vi "OpenSubVIS.vi"(8 "error in (no error)":errorcluster caption="错误输入（无错误）", 10 "自动关闭前面板？":bool, 11 "路径或VI名称":path) -> (0 "error out":errorcluster caption="错误输出")   [LabVIEW 2018]
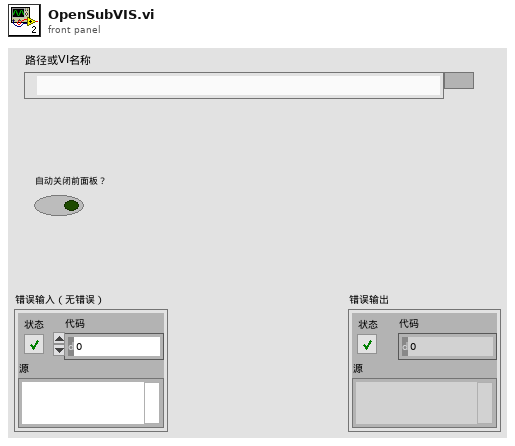
[diagram p1: front panel]
types:
  T1 = enum32{"Bad", "Idle", "Run top level", "Running"}
  T2 = enum32{"Invalid", "Standard", "Closed", "Hidden", "Minimized", "Maximized"}
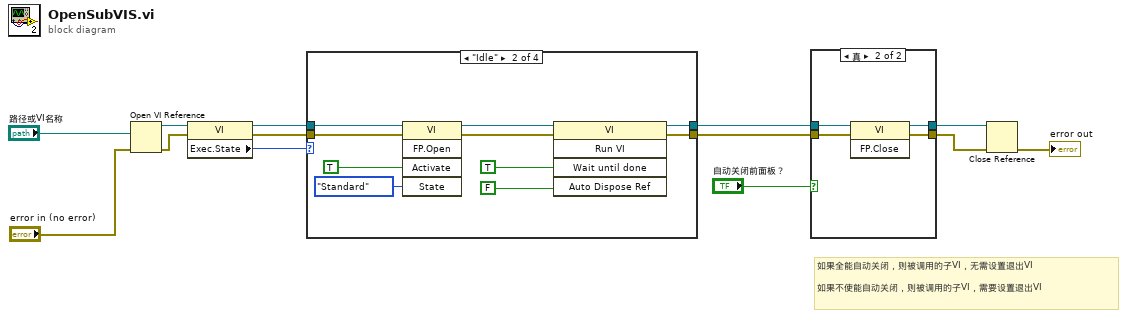
[diagram p0: block diagram]
diagram:
  # "如果全能自动关闭，则被调用的子VI，无需设置退出VI\n\n如果不使能自动关闭，则被调用的子VI，需要设置退出VI"
  n1 = Open VI Reference(vi path="路径或VI名称", error in (no error)="error in (no error)") -> (vi reference=w13:refnum<vi>, error out=w8:errorcluster)  [unwired: 4 in]
  n2 = property class="VI"(reference=w13, error in=w8) -> (reference out=w10:refnum<vi>, error out=w9:errorcluster, "Exec.State"=w11:T1)
  n3 = case shown="\"Idle\"" w11 {
    tunnel: w10 -> [w15 w25 w27 w29]
    tunnel: w9 -> [w14 w22 w26 w28]
    tunnel: [w15 w17 w27 w29] -> w5
    tunnel: [w14 w16 w26 w28] -> w4
    frame "Bad", Default {
    }
    frame "Idle" {
      n4 = invoke class="VI" method="FP.Open"(reference=w25, error in=w22, "Activate"=TRUE ("结束前等待"), "State"=T2."Standard" ("状态")) -> (reference out=w24:refnum<vi>, error out=w23:errorcluster)  [unwired: 1 in, 3 out]
      n5 = invoke class="VI" method="Run VI"(reference=w24, error in=w23, "Wait until done"=TRUE, "Auto Dispose Ref"=FALSE) -> (reference out=w17:refnum<vi>, error out=w16:errorcluster)  [unwired: 1 in, 3 out]
    }
    frame "Run top level" {
    }
    frame "Running" {
    }
  }
  n6 = case shown="真" "自动关闭前面板？" {
    tunnel: w5 -> [w31 w35]
    tunnel: w4 -> [w30 w34]
    tunnel: [w31 w33] -> w3
    tunnel: [w30 w32] -> w2
    frame False {
    }
    frame True {
      n7 = invoke class="VI" method="FP.Close"(reference=w35, error in=w34) -> (reference out=w33:refnum<vi>, error out=w32:errorcluster)  [unwired: 1 in, 1 out]
    }
  }
  n8 = Close Reference(reference=w3, error in (no error)=w2) -> (error out=→"error out":errorcluster)
